vi "FFTKundtsTube.vi"() -> ()   [LabVIEW 2014]
uses:
  <vilib>/express/express analysis/Spectral/Block/exnSpectralBlock spectral measurements RMS poly.vi
  <vilib>/express/express analysis/Spectral/Block/exnSpectralBlock spectral measurements RMS WFM.vi
  <vilib>/express/express analysis/Spectral/XNode/ExpressSpectralMeasurementsBlockNode.xnode
panel:
  in  "Time (s)":dbl
  out "Waveform Graph":cluster{"f0":dbl, "df":dbl, "magnitude":dbl[]}(graph)
  in  "stop":bool
  in  "Averages":dbl
  in  "Rate":dbl
  in  "error in":errorcluster
  out "error out":errorcluster
  out "data":dynamicdata(graph)
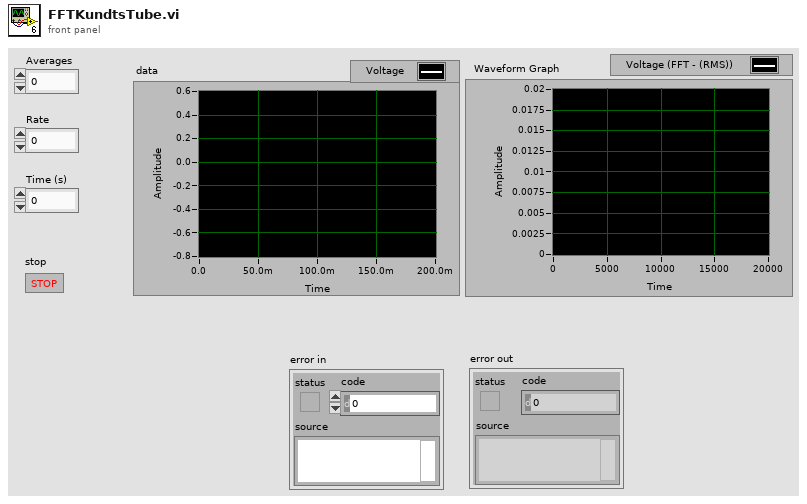
[diagram p1: front panel]
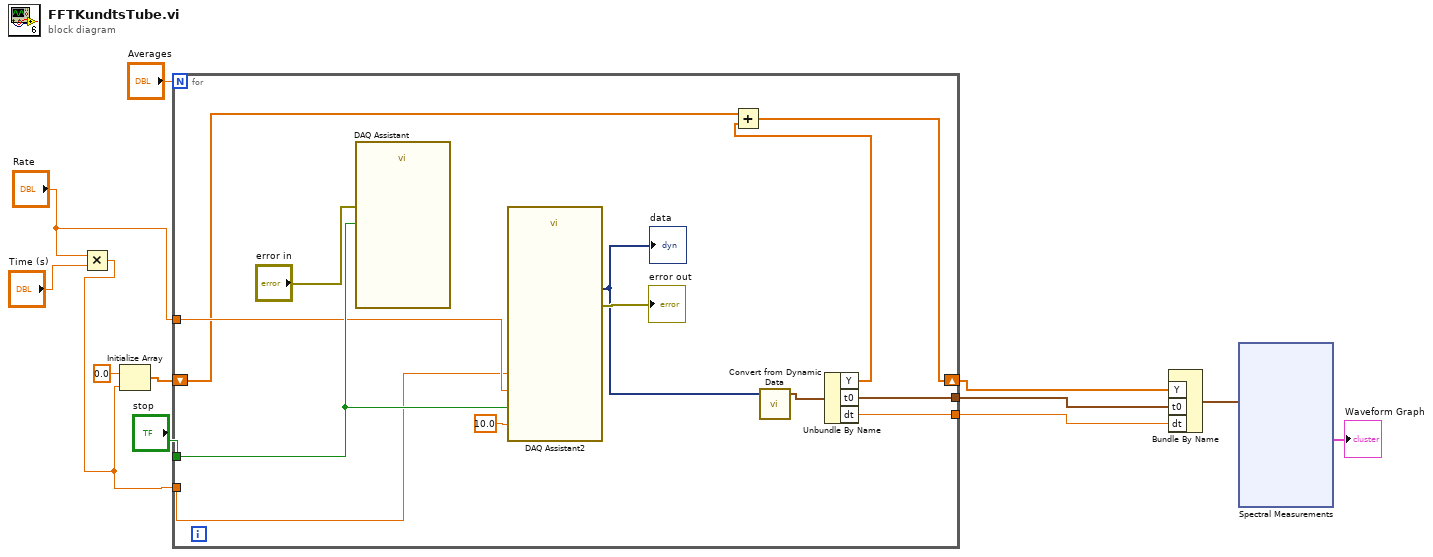
[diagram p0: block diagram]
diagram:
  n1 = Multiply(x="Rate", y="Time (s)") -> (x*y=w1:dbl)
  n2 = Initialize Array(0.0 ("element"), w1) -> (w6:dbl[])
  n3 = for {
    N: "Averages" -> [_]
    tunnel: "Rate" -> [w22]
    tunnel: "stop" -> [w23]
    tunnel: w1 -> [w20]
    shift-right: [w13] -> w4
    shift-left: w6 -> [w15]
    tunnel: [w18] -> w9
    tunnel: [w17] -> w8
    n4 = call "DAQ Assistant"("error in"="error in", "stop (T)"=w23) -> ()  [unwired: 16 in, 2 out]
    n5 = call "DAQ Assistant2"("rate"=w22, "number of samples"=w20, "timeout (s)"=10.0, "stop (T)"=w23) -> ("data"=w14:dynamicdata, "error out"=→"error out":errorcluster)  [unwired: 13 in, 1 out]
    "data" <- w14
    n6 = call "Convert from Dynamic Data"("Dynamic Data Type"=w14) -> ("Waveform"=w19:waveform(dbl))  [unwired: 3 in]
    n7 = Unbundle By Name(w19) -> ("Y"=w16:dbl[], "t0"=w18:timestamp, "dt"=w17:dbl)
    n8 = Add(x=w15, y=w16) -> (x+y=w13:dbl[])
  }
  n9 = Bundle By Name("Y"=w4, "t0"=w9, "dt"=w8) -> (w7:waveform(dbl))  [unwired: 1 in]
  n10 = xnode "Spectral Measurements"("Signals"=w7) -> ("FFT - (RMS)"=→"Waveform Graph":cluster{"f0":dbl, "df":dbl, "magnitude":dbl[]})  [unwired: 1 in, 2 out]
